vi "absAngle.vi"(4 "Numeric":dbl) -> (1 "Numeric 2":dbl)   [LabVIEW 2016]
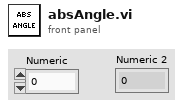
[diagram p1: front panel]
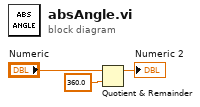
[diagram p0: block diagram]
diagram:
  n1 = Quotient & Remainder(x="Numeric", y=360.0) -> (x-y*floor(x/y)=→"Numeric 2":dbl)  [unwired: 1 out]
